vi "Division.vi"() -> ()   [LabVIEW 2014]
panel:
  out "Result":dbl
  in  "Num 2":dbl
  in  "Num 1":dbl
  # "Click          to run"
  # "÷"
  # "="
  # "Division"
  # "The goal of this exercise is simple. Make a calculator that does division. The challenge is that you cannot use the built in divide (or multiply) functions from the mathematics pallete. \n\nFurthermore, you must calculate the quotient to four decimal places."
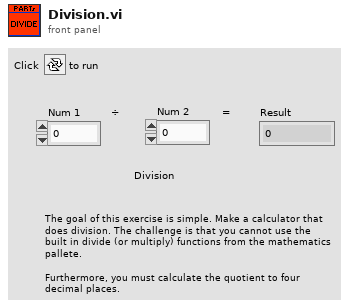
[diagram p1: front panel]
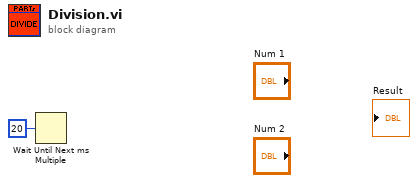
[diagram p0: block diagram]
diagram:
  n1 = Wait Until Next ms Multiple(millisecond multiple=u32 20) -> ()  [unwired: 1 out]
